vi "BuildFieldArray.vi"(1 "Step Size (mT)":dbl format="%#_13g", 2 "Field Amplitude (mT)":dbl format="%#_13g") -> (0 "Field Array":dbl[](array[numeric]))   [LabVIEW 2016]
panel:
  out "size(s)":i32
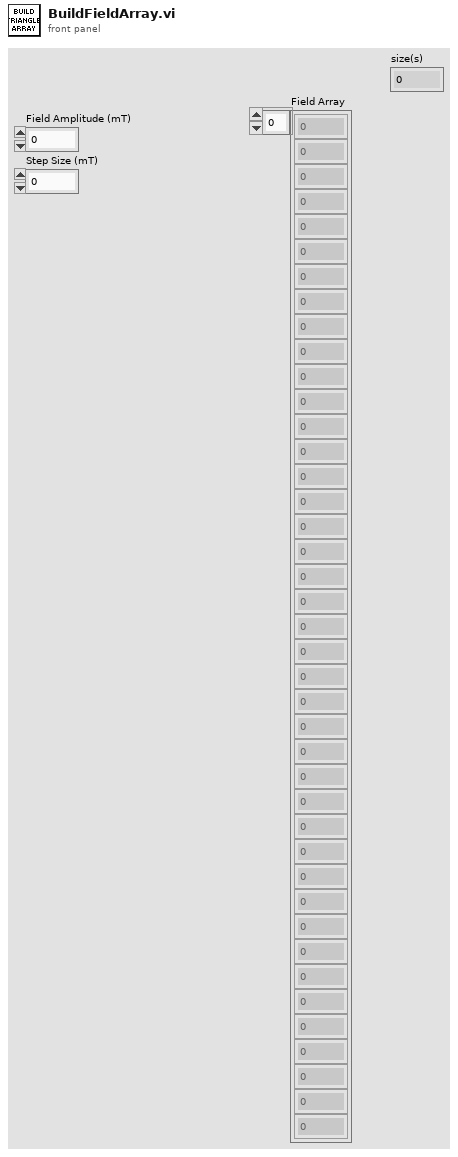
[diagram p1: front panel]
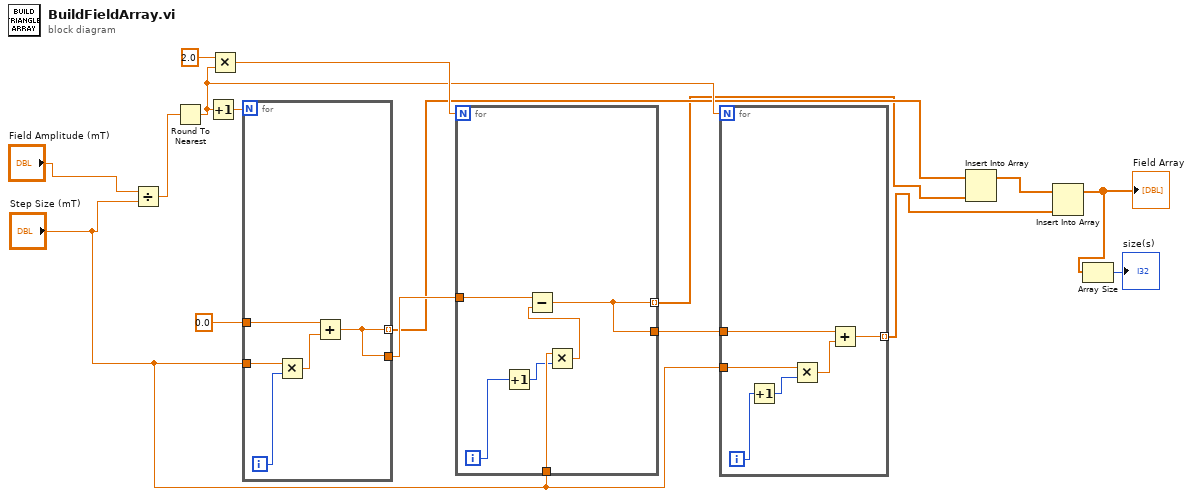
[diagram p0: block diagram]
diagram:
  n1 = Divide(x="Field Amplitude (mT)", y="Step Size (mT)") -> (x/y=w15:dbl)
  n2 = Round To Nearest(number=w15) -> (nearest integer value=w9:dbl)
  n3 = Increment(x=w9) -> (x+1=w14:dbl)
  n4 = Multiply(x=2.0, y=w9) -> (x*y=w11:dbl)
  n5 = for {
    N: w14 -> [_]
    tunnel: "Step Size (mT)" -> [w19]
    tunnel: 0.0 -> [w18]
    tunnel: [w17] -> w6 mode=indexing
    tunnel: [w17] -> w10
    i -> [w20]
    n6 = Multiply(x=w19, y=w20) -> (x*y=w21:dbl)
    n7 = Add(x=w18, y=w21) -> (x+y=w17:dbl)
  }
  n8 = for {
    N: w11 -> [_]
    tunnel: "Step Size (mT)" -> [w26]
    tunnel: w10 -> [w24]
    tunnel: [w22] -> w5 mode=indexing
    tunnel: [w22] -> w7
    i -> [w27]
    n9 = Increment(x=w27) -> (x+1=w25:i32)
    n10 = Multiply(x=w26, y=w25) -> (x*y=w23:dbl)
    n11 = Subtract(x=w24, y=w23) -> (x-y=w22:dbl)
  }
  n12 = for {
    N: w9 -> [_]
    tunnel: "Step Size (mT)" -> [w32]
    tunnel: w7 -> [w30]
    tunnel: [w28] -> w3 mode=indexing
    i -> [w31]
    n13 = Increment(x=w31) -> (x+1=w33:i32)
    n14 = Multiply(x=w32, y=w33) -> (x*y=w29:dbl)
    n15 = Add(x=w30, y=w29) -> (x+y=w28:dbl)
  }
  n16 = Insert Into Array(array=w6, new element=w5) -> (w4:dbl[])  [unwired: 1 in]
  n17 = Insert Into Array(array=w4, new element=w3) -> (w2:dbl[])  [unwired: 1 in]
  "Field Array" <- w2
  n18 = Array Size(array=w2) -> (size(s)=→"size(s)":i32)
